vi "Config Curve Header.vi"(0 "VISA resource name":refnum<visa-resource-name>, 1 "Curve Data Format (V/K:0)":u16(ring) items=["V/K", "Ohms/K", "Log Ohms/K"], 2 "Temp Coefficient (Neg:0)":u16(ring) items=["Negative", "Positive"], 5 "Curve (21)":dbl=21.0 min=21.0 max=28.0 step=1.0, 7 "Curve Name (\"\")":string, 9 "Curve Serial Number (\"\")":string, 11 "error in (no error)":errorcluster, 12 "Limit Value (475.00)":dbl=475.0 min=0.0 max=999.99 step=0.01 format="%.2f") -> (4 "VISA resource name out":refnum<visa-resource-name>, 15 "error out":errorcluster)   [LabVIEW 2012, in "Lake Shore Cryotronics 218.lvlib"]
doc: "This VI Configures a user curve header."
uses:
  <instrlib>/Lake Shore Cryotronics 218/Lake Shore Cryotronics 218.lvlib
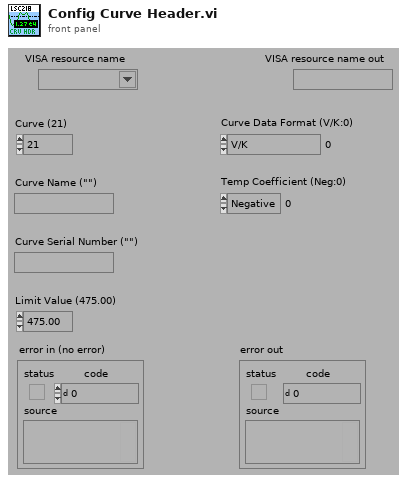
[diagram p1: front panel]
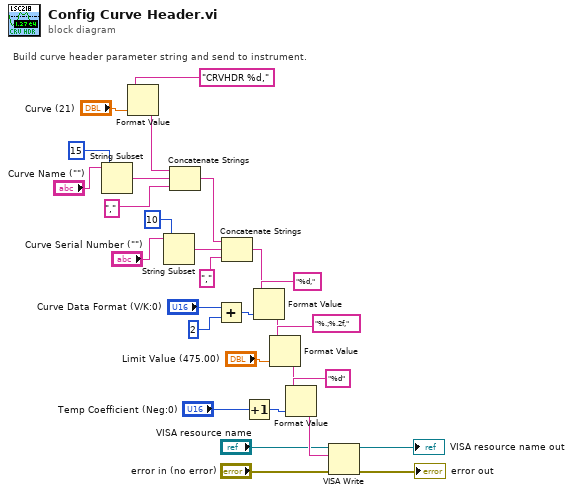
[diagram p0: block diagram]
diagram:
  # "Build curve header parameter string and send to instrument."
  n1 = String Subset(string="Curve Name (\"\")", length (rest)=15) -> (substring=w24:string)  [unwired: 1 in]
  n2 = Format Value(format string="CRVHDR %d,", value (0)="Curve (21)") -> (output string=w25:string)  [unwired: 1 in]
  n3 = String Subset(string="Curve Serial Number (\"\")", length (rest)=10) -> (substring=w28:string)  [unwired: 1 in]
  n4 = Concatenate Strings(w25, w24, ",") -> (w29:string)
  n5 = Add(x="Curve Data Format (V/K:0)", y=u16 2) -> (x+y=w5:u16)
  n6 = Concatenate Strings(w29, w28, ",") -> (w16:string)
  n7 = Increment(x="Temp Coefficient (Neg:0)") -> (x+1=w14:u16)
  n8 = Format Value(string ("")=w16, format string="%d,", value (0)=w5) -> (output string=w18:string)
  n9 = Format Value(string ("")=w18, format string="%.;%.2f,", value (0)="Limit Value (475.00)") -> (output string=w12:string)
  n10 = Format Value(string ("")=w12, format string="%d", value (0)=w14) -> (output string=w8:string)
  n11 = VISA Write(VISA resource name="VISA resource name", write buffer=w8, error in (no error)="error in (no error)") -> (VISA resource name out=→"VISA resource name out":refnum<visa-resource-name>, error out=→"error out":errorcluster)  [unwired: 1 out]
